vi "SetAdOff.vi"(0 "pos":bool=TRUE, 1 "Offset":u8) -> ()   [LabVIEW 2014]
uses:
  ESLSCDLL.dll
panel:
  # "neg"
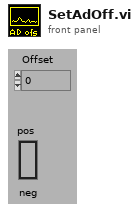
[diagram p1: front panel]
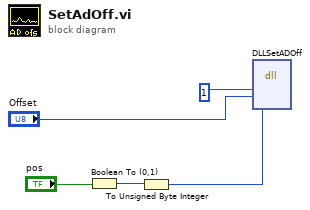
[diagram p0: block diagram]
diagram:
  n1 = Boolean To (0,1)(Boolean="pos") -> (0, 1=w2:i16)
  n2 = To Unsigned Byte Integer(number=w2) -> (unsigned 8bit integer=w1:u8)
  n3 = dll-call lib="C:/Users/Gerhard/Documents/New64/lv/1cam/board.vis/ESLSCDLL.dll" fn="DLLSetADOff"("drv"=u32 1, "ofs"="Offset", "pos"=w1) -> ()  [unwired: 7 in, 2 out]
